vi "get image ROI.vi"(8 "error in (no error)":errorcluster, 10 "data folder Path":path, 11 "DAQOrcaFlash in":refnum<class "DAQOrcaFlash.lvclass">) -> (0 "error out":errorcluster, 2 "Array":i32[][](array[numeric]), 3 "DAQOrcaFlash out":refnum<class "DAQOrcaFlash.lvclass">)   [LabVIEW 2012, in "DAQOrcaFlash.lvclass"]
uses:
  DAQOrcaFlash.lvclass
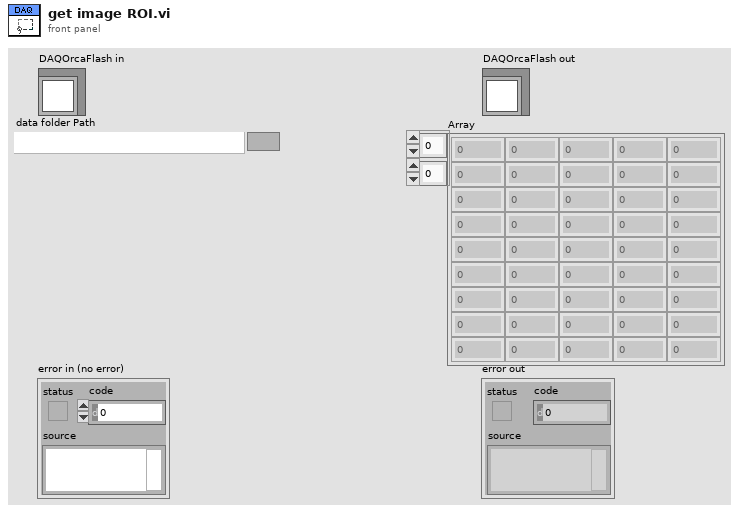
[diagram p1: front panel]
types:
  T1 = typedef "Image Type" = u32
  T2 = typedef "IMAQ Image.ctl" = refnum<image>
  T3 = typedef "ROI Descriptor" = cluster{"Global Rectangle":i32[], "Contours":cluster{"ID":enum32{"External", "Internal"}, "Type":u32, "Coordinates":i32[]}[]}
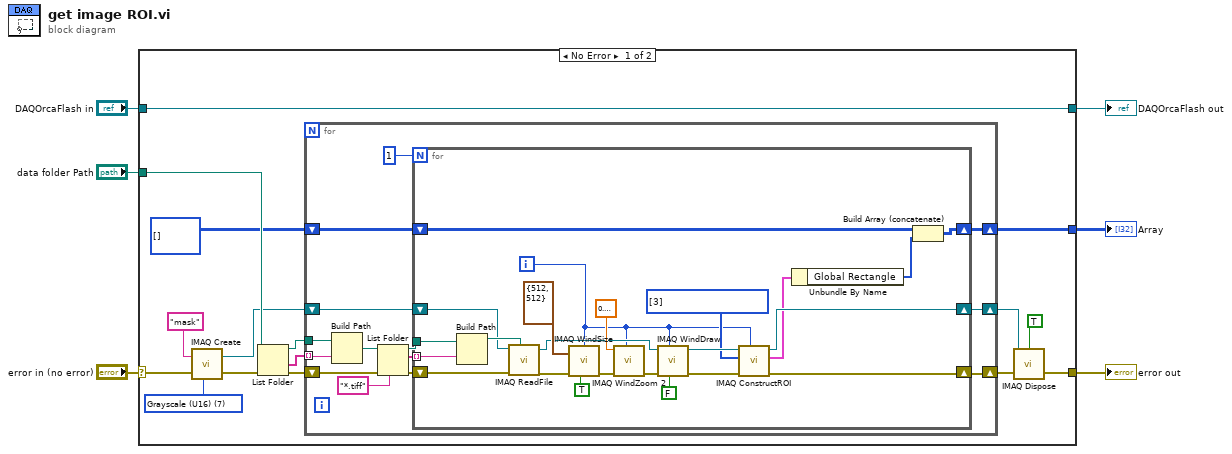
[diagram p0: block diagram]
diagram:
  n1 = case shown="No Error" "error in (no error)" {
    selector: "error in (no error)" -> [w17 w61]
    tunnel: [w11 w61] -> w5
    tunnel: [w22 w60] -> w3
    tunnel: "DAQOrcaFlash in" -> [w22 w60]
    tunnel: "data folder Path" -> [w19 _]
    tunnel: [w7 _] -> w1
    frame No Error {
      w14 = T1 7 items=["Grayscale (U8)", "Grayscale (I16)", "Grayscale (SGL)", "Complex (CSG)", "RGB (U32)", "HSL (U32)", "RGB (U64)", "Grayscale (U16)"] ("Image Type")
      n2 = call "IMAQ Create"("Image Name"="mask", "Image Type"=w14, "error in (no error)"=w17) -> ("New Image"=w13:T2, "error out"=w16:errorcluster)  [unwired: 2 in]
      n3 = List Folder(path=w19, error in=w16) -> (path out=w18:path, folder names=w20:string[], error out=w21:errorcluster)  [unwired: 2 in, 1 out]
      n4 = for {
        shift-right: [w25] -> w12
        shift-left: w21 -> [w34]
        tunnel: w20 -> [w35] mode=indexing
        tunnel: w18 -> [w36]
        shift-right: [w26] -> w10
        shift-left: w13 -> [w27]
        shift-right: [w23] -> w7
        shift-left: i32[][] [] -> [w24]
        n5 = Build Path(base path=w36, name or relative path=w35) -> (appended path=w33:path)
        n6 = List Folder(path=w33, pattern="*.tiff", error in=w34) -> (path out=w28:path, filenames=w30:string[], error out=w31:errorcluster)  [unwired: 1 in, 1 out]
        n7 = for {
          N: 1 -> [_]
          tunnel: w30 -> [w59] mode=indexing
          tunnel: w28 -> [w58]
          shift-right: [w41] -> w26
          shift-left: w27 -> [w55]
          shift-right: [w45] -> w25
          shift-left: w31 -> [w57]
          shift-right: [w37] -> w23
          shift-left: w24 -> [w39]
          i -> [w42]
          w43 = u32[] [3] items=["No Selection", "Point", "Line", "Rectangle", "Oval", "Polygon", "Freehand Region", "Annulus", "Zoom", "Pan", "Broken Line", "Freehand Line", "Rotated Rectangle"] ("Tools")
          n8 = Build Path(base path=w58, name or relative path=w59) -> (appended path=w56:path)
          n9 = call "IMAQ ReadFile"("File Path"=w56, "error in (no error)"=w57, "Image"=w55) -> ("error out"=w49:errorcluster, "Image Out"=w47:T2)  [unwired: 4 in, 3 out]
          n10 = call "IMAQ WindSize"("error in (no error)"=w49, "Get/Set Status? (Set)"=TRUE, "Width & Height"=cluster{"Width":i32, "Height":i32} {"Width"=512, "Height"=512}, "Window Number"=w42) -> ("error out"=w53:errorcluster)  [unwired: 2 in, 2 out]
          n11 = call "IMAQ WindZoom 2"("Window Number (0...15)"=w42, "error in (no error)"=w53, "Zoom Factor"=sgl 0.2) -> ("error out"=w52:errorcluster)  [unwired: 5 in, 3 out]
          n12 = call "IMAQ WindDraw"("Resize to Image Size? (Y)"=FALSE, "Window Number (0...15)"=w42, "error in (no error)"=w52, "Image"=w47) -> ("error out"=w46:errorcluster, "Image Out (duplicate)"=w44:T2)  [unwired: 6 in]
          n13 = call "IMAQ ConstructROI"("Window Number (-1...15)"=w42, "error in (no error)"=w46, "Tools"=w43, "Image"=w44) -> ("error out"=w45:errorcluster, "ROI Descriptor Out"=w40:T3, "Image Out (duplicate)"=w41:T2)  [unwired: 4 in, 1 out]
          n14 = Unbundle By Name(w40) -> ("Global Rectangle"=w38:i32[])
          n15 = Build Array (concatenate)(w39, w38) -> (w37:i32[][])
        }
      }
      n16 = call "IMAQ Dispose"("All Images? (No)"=TRUE, "Image"=w10, "error in (no error)"=w12) -> ("error out"=w11:errorcluster)  [unwired: 3 in]
    }
    frame Error {
    }
  }
  "error out" <- w5
  "DAQOrcaFlash out" <- w3
  "Array" <- w1
